vi "电源管理UI.vi"() -> ()   [LabVIEW 2016, in "PLC.lvlib"]
uses:
  PLC.lvlib
  <vilib>/Utility/miscctls.llb/LVPointTypeDef.ctl
  <vilib>/ptbypt/NI_PtbyPt.lvlib
panel:
  in  "副屏看门狗启用":u16(ring) caption="副屏看门狗启用：" items=["关闭", "打开"]
  in  "副屏看门狗设置":u16 caption="副屏看门狗设置："
  out "副屏看门狗计时":u16 caption="副屏看门狗计时："
  in  "主屏看门狗启用":u16(ring) caption="主屏看门狗启用：" items=["关闭", "打开"]
  in  "主屏看门狗设置":u16 caption="主屏看门狗设置："
  out "主屏看门狗计时":u16 caption="主屏看门狗计时："
  out "漏电报警累加值":u16 caption="漏电报警累加值："
  out "外部电源状态":u16(ring) caption="外部电源状态：" items=["正常", "异常"]
  out "当前报警状态":u16(ring) caption="当前报警状态：" items=["无报警"=0, "过压报警"=1, "欠压报警"=2, "过流报警"=4, "漏电报警"=8]
  out "通讯状态":u16(ring) caption="通讯状态：" items=["正常", "异常"]
  out "合闸状态":u16(ring) caption="内部电源状态：" items=["断开", "打开"]
  out "过流报警累加值":u16 caption="过流报警累加值："
  out "欠压报警累加值":u16 caption="欠压报警累加值："
  out "过压报警累加值":u16 caption="过压报警累加值："
  out "当前漏电电流":dbl caption="当前漏电电流："
  out "当前电流":dbl caption="当前电流："
  out "当前电压":u16 caption="当前电压："
  in  "总氮电源":bool
  in  "CODCr电源":bool
  in  "总磷电源":bool
  in  "氨氮电源":bool
  in  "CODMn电源":bool
  in  "多参数电源":bool
  # "s"
  # "s"
  # "s"
  # "s"
  # "mA"
  # "A"
  # "V"
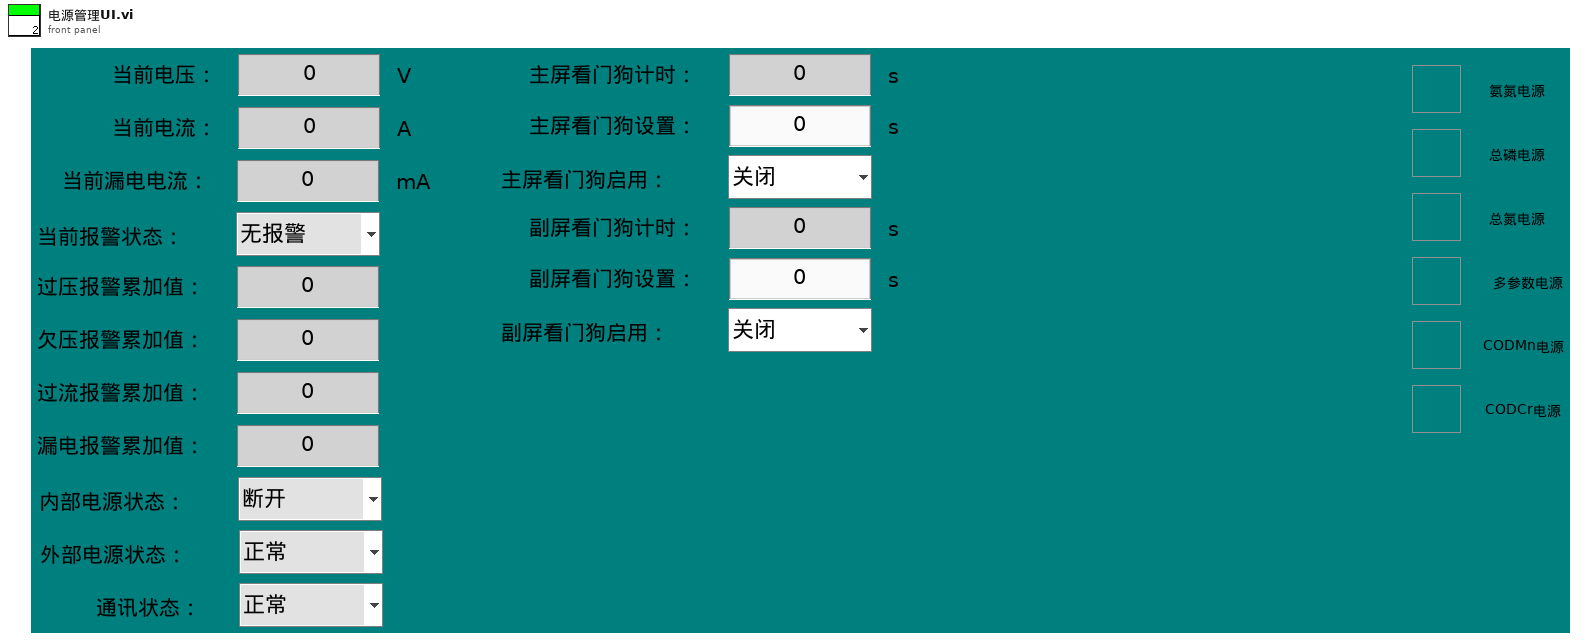
[diagram p1: front panel]
types:
  T1 = typedef "LVPointTypeDef.ctl" = cluster{"Horizontal":i16, "Vertical":i16}
  T2 = cluster{"R0":i16, "R1":i16, "R2":i16, "R3":i16, "R4":i16, "R5":i16, "R6":i16, "R7":i16, "R8":i16, "R9":i16, "R10":i16, "R11":i16, "R12":i16, "R13":i16, "R14":i16, "R15":i16, "R16":i16, "R17":i16, "R18":i16, "R19":i16, "R20":i16, "R21":i16, "R22":i16, "R23":i16, "R24":i16, "R25":i16, "R26":i16, "R27":i16, "R28":i16, "R29":i16, "R30":i16, "R31":i16, "R32":i16, "R33":i16, "R34":i16, "R35":i16, "R36":i16, "R37":i16, "R38":i16, "R39":i16}
  T3 = cluster{"R100":i16, "R101":i16, "R102":i16, "R103":i16, "R104":i16, "R105":i16, "R106":i16, "R107":i16, "R108":i16, "R109":i16, "R110":i16, "R111":i16, "R112":i16, "R113":i16, "R114":i16, "R115":i16, "R116":i16, "R117":i16, "R118":i16, "R119":i16}
  T4 = cluster{"时间标识":timestamp, "设备":string, "日志信息":string}
  T5 = cluster{"命令":string, "数据":cluster{"starting address":u16, "holding register values":u16[]}}
  T6 = cluster{"命令":string, "数据":cluster{"starting address":u16, "holding register value":u16}}
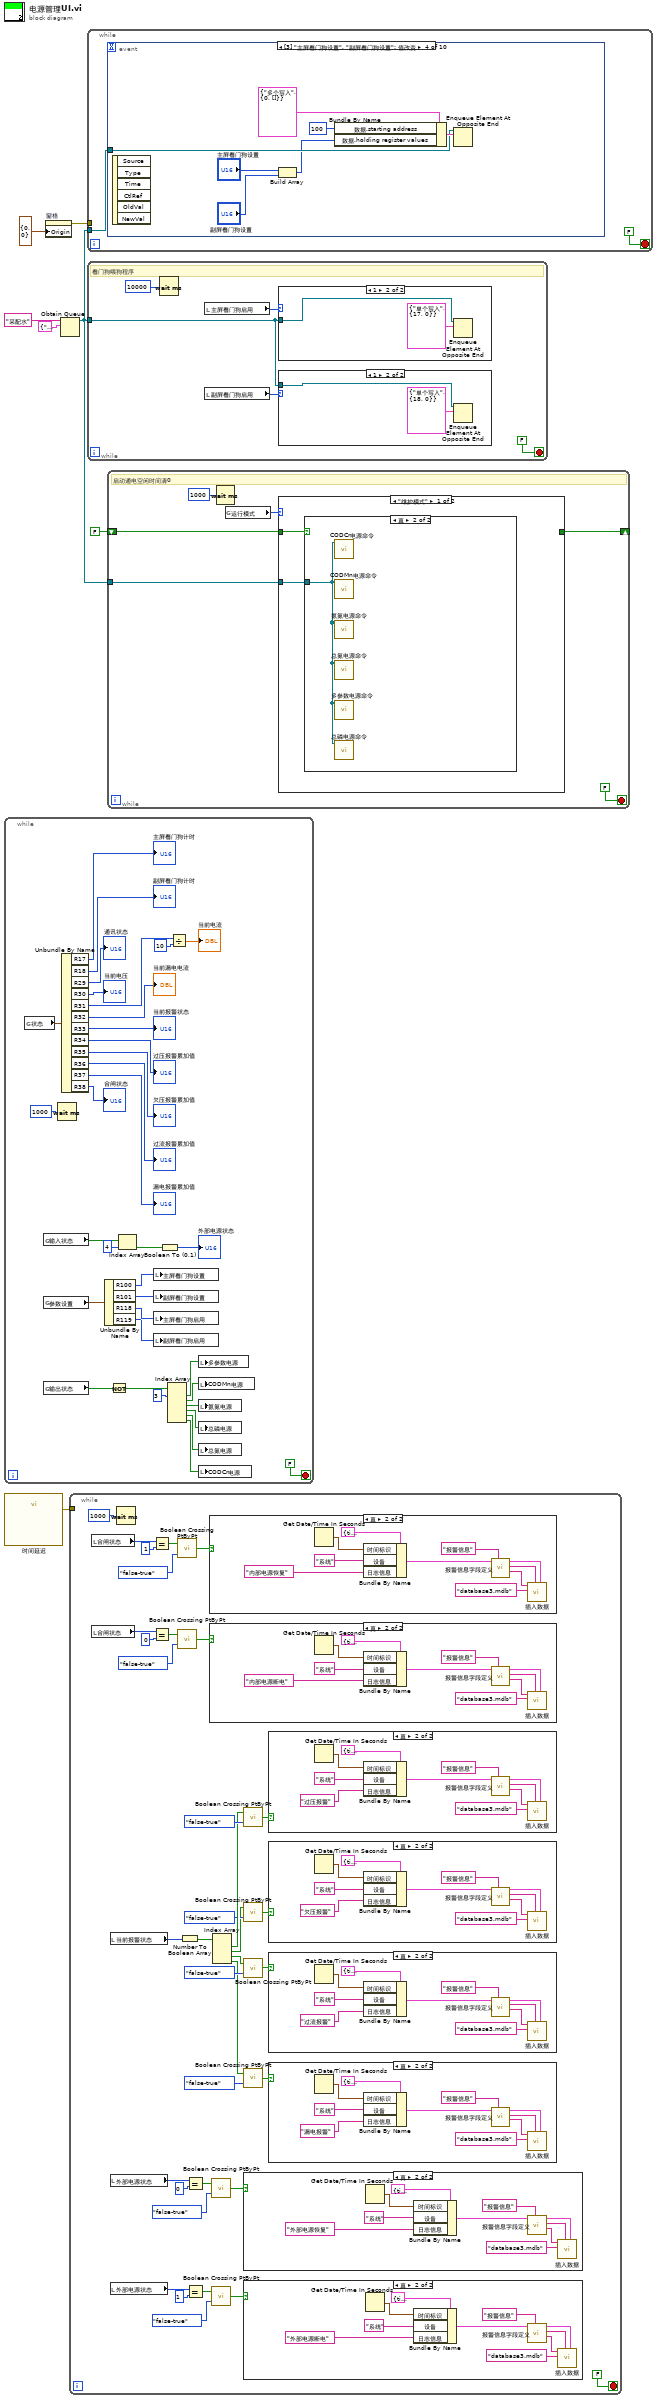
[diagram p0: block diagram]
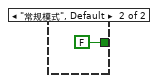
[diagram p13: hidden frame]
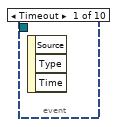
[diagram p14: hidden frame]
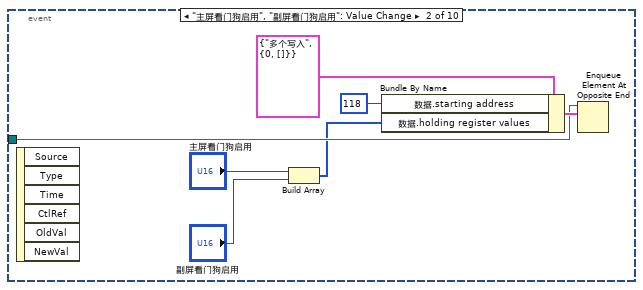
[diagram p15: hidden frame]
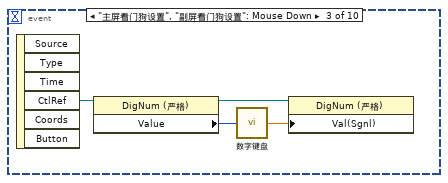
[diagram p16: hidden frame]
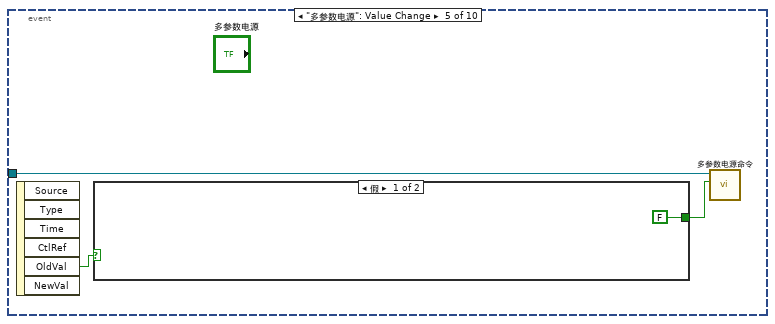
[diagram p17: hidden frame]
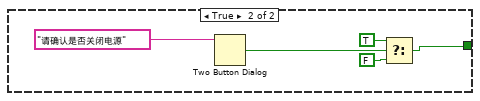
[diagram p18: hidden frame]
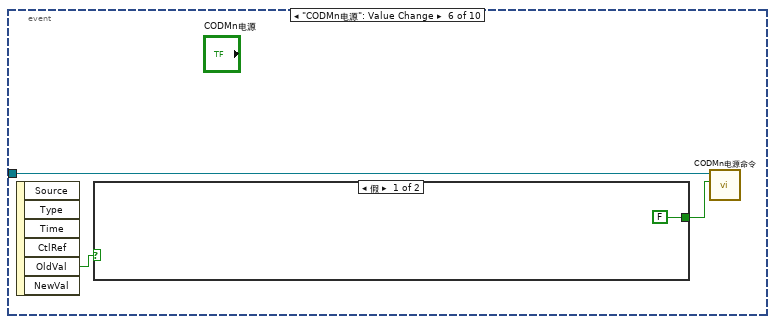
[diagram p19: hidden frame]
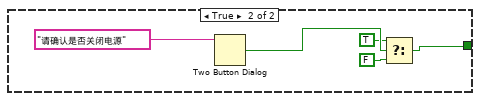
[diagram p20: hidden frame]
diagram:
  n1 = while {
    stop <- FALSE stop-if-true
    n2 = global read "采配水全局变量.vi" "状态"() -> (w31:T2)
    n3 = global read "采配水全局变量.vi" "输入状态"() -> (w18:bool[])
    n4 = global read "采配水全局变量.vi" "参数设置"() -> (w12:T3)
    n5 = global read "采配水全局变量.vi" "输出状态"() -> (w40:bool[])
    n6 = Wait (ms)(milliseconds to wait=u32 1000 ("等待时间（毫秒）")) -> ()  [unwired: 1 out]
    n7 = Unbundle By Name(w31) -> ("R17"=→"主屏看门狗计时":i16, "R18"=→"副屏看门狗计时":i16, "R29"=→"通讯状态":i16, "R30"=→"当前电压":i16, "R31"=w28:i16, "R32"=→"当前漏电电流":i16, "R33"=→"当前报警状态":i16, "R34"=→"过压报警累加值":i16, "R35"=→"欠压报警累加值":i16, "R36"=→"过流报警累加值":i16, "R37"=→"漏电报警累加值":i16, "R38"=→"合闸状态":i16)
    n8 = Unbundle By Name(w12) -> ("R100"=w11:i16, "R101"=w10:i16, "R118"=w9:i16, "R119"=w8:i16)
    n9 = Not(x=w40) -> (.not. x?=w32:bool[])
    n10 = Index Array(array=w18, index=4 ("索引")) -> (element=w16:bool)
    n11 = local write "主屏看门狗设置"(w11) -> ()
    n12 = local write "副屏看门狗设置"(w10) -> ()
    n13 = local write "主屏看门狗启用"(w9) -> ()
    n14 = local write "副屏看门狗启用"(w8) -> ()
    n15 = Boolean To (0,1)(Boolean=w16) -> (0, 1=→"外部电源状态":i16)
    n16 = Index Array(array=w32, index #1=3 ("索引")) -> (element #1=w35:bool, element #2=w38:bool, element #3=w37:bool, element #4=w36:bool, element #5=w34:bool, element #6=w33:bool)  [unwired: 5 in]
    n17 = Divide(x=w28, y=i16 10) -> (x/y=→"当前电流":dbl)
    n18 = local write "多参数电源"(w35) -> ()
    n19 = local write "CODMn电源"(w38) -> ()
    n20 = local write "氨氮电源"(w37) -> ()
    n21 = local write "总磷电源"(w36) -> ()
    n22 = local write "总氮电源"(w34) -> ()
    n23 = local write "CODCr电源"(w33) -> ()
  }
  n24 = call "时间延迟"() -> ("error out"=w2:errorcluster)  [unwired: 11 in]
  n25 = property on="窗格" class="Pane"("Origin"=T1 {"Horizontal"=0, "Vertical"=0} ("原点")) -> (error out=w4:errorcluster)  [unwired: 2 in, 1 out]
  n26 = Obtain Queue(name (unnamed)="采配水" ("名称（未命名）"), element data type=cluster{"命令":string, "数据":variant} {"命令"="", "数据"=variant}) -> (queue out=w1:refnum<queue>)  [unwired: 3 in, 2 out]
  n27 = while {
    tunnel: w2 -> [_]
    stop <- FALSE stop-if-true
    n28 = local read "合闸状态"() -> (w68:u16)
    n29 = local read "合闸状态"() -> (w59:u16)
    n30 = local read "当前报警状态"() -> (w58:u16)
    n31 = local read "外部电源状态"() -> (w78:u16)
    n32 = local read "外部电源状态"() -> (w69:u16)
    n33 = Wait (ms)(milliseconds to wait=u32 1000 ("等待时间（毫秒）")) -> ()  [unwired: 1 out]
    n34 = Equal?(x=w68, y=u16 1) -> (x = y?=w66:bool)
    n35 = Equal?(x=w59, y=u16 0) -> (x = y?=w61:bool)
    n36 = call <vilib>:"Boolean Crossing PtByPt.vi"("direction"=enum16{"either", "false-true", "true-false"}."false-true", "input"=w66) -> ("crossing"=w64:bool)  [unwired: 1 in]
    n37 = call <vilib>:"Boolean Crossing PtByPt.vi"("direction"=enum16{"either", "false-true", "true-false"}."false-true", "input"=w61) -> ("crossing"=w63:bool)  [unwired: 1 in]
    n38 = Number To Boolean Array(number=w58) -> (Boolean array=w57:bool[])
    n39 = Equal?(x=w78, y=u16 0) -> (x = y?=w76:bool)
    n40 = Equal?(x=w69, y=u16 1) -> (x = y?=w71:bool)
    n41 = case shown="真" w64 {
      frame False {
      }
      frame True {
        n42 = Get Date/Time In Seconds() -> (seconds since 1Jan1904=w137:timestamp)
        n43 = Bundle By Name(cluster=T4 {"时间标识"=timestamp(0 s since 1904-01-01), "设备"="", "日志信息"=""} ("data in"), "时间标识"=w137, "设备"="系统", "日志信息"="内部电源恢复") -> (w136:T4)
        n44 = call "报警信息字段定义.vi"("table输入"="报警信息", "data in"=w136) -> ("table输出"=w132:string, "columns"=w131:string[], "data out"=w130:T4)  [unwired: 7 in]
        n45 = call "插入数据.vi"("data"=w130, "columns"=w131, "database"="database3.mdb", "table"=w132) -> ()  [unwired: 7 in, 1 out]
      }
    }
    n46 = case shown="真" w63 {
      frame False {
      }
      frame True {
        n47 = Get Date/Time In Seconds() -> (seconds since 1Jan1904=w127:timestamp)
        n48 = Bundle By Name(cluster=T4 {"时间标识"=timestamp(0 s since 1904-01-01), "设备"="", "日志信息"=""} ("data in"), "时间标识"=w127, "设备"="系统", "日志信息"="内部电源断电") -> (w126:T4)
        n49 = call "报警信息字段定义.vi"("table输入"="报警信息", "data in"=w126) -> ("table输出"=w122:string, "columns"=w121:string[], "data out"=w120:T4)  [unwired: 7 in]
        n50 = call "插入数据.vi"("data"=w120, "columns"=w121, "database"="database3.mdb", "table"=w122) -> ()  [unwired: 7 in, 1 out]
      }
    }
    n51 = call <vilib>:"Boolean Crossing PtByPt.vi"("direction"=enum16{"either", "false-true", "true-false"}."false-true", "input"=w76) -> ("crossing"=w74:bool)  [unwired: 1 in]
    n52 = call <vilib>:"Boolean Crossing PtByPt.vi"("direction"=enum16{"either", "false-true", "true-false"}."false-true", "input"=w71) -> ("crossing"=w73:bool)  [unwired: 1 in]
    n53 = Index Array(array=w57) -> (element #1=w55:bool, element #2=w49:bool, element #3=w48:bool, element #4=w45:bool)  [unwired: 4 in]
    n54 = call <vilib>:"Boolean Crossing PtByPt.vi"("direction"=enum16{"either", "false-true", "true-false"}."false-true", "input"=w55) -> ("crossing"=w54:bool)  [unwired: 1 in]
    n55 = call <vilib>:"Boolean Crossing PtByPt.vi"("direction"=enum16{"either", "false-true", "true-false"}."false-true", "input"=w49) -> ("crossing"=w53:bool)  [unwired: 1 in]
    n56 = call <vilib>:"Boolean Crossing PtByPt.vi"("direction"=enum16{"either", "false-true", "true-false"}."false-true", "input"=w48) -> ("crossing"=w50:bool)  [unwired: 1 in]
    n57 = call <vilib>:"Boolean Crossing PtByPt.vi"("direction"=enum16{"either", "false-true", "true-false"}."false-true", "input"=w45) -> ("crossing"=w47:bool)  [unwired: 1 in]
    n58 = case shown="真" w74 {
      frame False {
      }
      frame True {
        n59 = Get Date/Time In Seconds() -> (seconds since 1Jan1904=w157:timestamp)
        n60 = Bundle By Name(cluster=T4 {"时间标识"=timestamp(0 s since 1904-01-01), "设备"="", "日志信息"=""} ("data in"), "时间标识"=w157, "设备"="系统", "日志信息"="外部电源恢复") -> (w156:T4)
        n61 = call "报警信息字段定义.vi"("table输入"="报警信息", "data in"=w156) -> ("table输出"=w152:string, "columns"=w151:string[], "data out"=w150:T4)  [unwired: 7 in]
        n62 = call "插入数据.vi"("data"=w150, "columns"=w151, "database"="database3.mdb", "table"=w152) -> ()  [unwired: 7 in, 1 out]
      }
    }
    n63 = case shown="真" w73 {
      frame False {
      }
      frame True {
        n64 = Get Date/Time In Seconds() -> (seconds since 1Jan1904=w147:timestamp)
        n65 = Bundle By Name(cluster=T4 {"时间标识"=timestamp(0 s since 1904-01-01), "设备"="", "日志信息"=""} ("data in"), "时间标识"=w147, "设备"="系统", "日志信息"="外部电源断电") -> (w146:T4)
        n66 = call "报警信息字段定义.vi"("table输入"="报警信息", "data in"=w146) -> ("table输出"=w142:string, "columns"=w141:string[], "data out"=w140:T4)  [unwired: 7 in]
        n67 = call "插入数据.vi"("data"=w140, "columns"=w141, "database"="database3.mdb", "table"=w142) -> ()  [unwired: 7 in, 1 out]
      }
    }
    n68 = case shown="真" w54 {
      frame False {
      }
      frame True {
        n69 = Get Date/Time In Seconds() -> (seconds since 1Jan1904=w117:timestamp)
        n70 = Bundle By Name(cluster=T4 {"时间标识"=timestamp(0 s since 1904-01-01), "设备"="", "日志信息"=""} ("data in"), "时间标识"=w117, "设备"="系统", "日志信息"="过压报警") -> (w116:T4)
        n71 = call "报警信息字段定义.vi"("table输入"="报警信息", "data in"=w116) -> ("table输出"=w112:string, "columns"=w111:string[], "data out"=w110:T4)  [unwired: 7 in]
        n72 = call "插入数据.vi"("data"=w110, "columns"=w111, "database"="database3.mdb", "table"=w112) -> ()  [unwired: 7 in, 1 out]
      }
    }
    n73 = case shown="真" w53 {
      frame False {
      }
      frame True {
        n74 = Get Date/Time In Seconds() -> (seconds since 1Jan1904=w107:timestamp)
        n75 = Bundle By Name(cluster=T4 {"时间标识"=timestamp(0 s since 1904-01-01), "设备"="", "日志信息"=""} ("data in"), "时间标识"=w107, "设备"="系统", "日志信息"="欠压报警") -> (w106:T4)
        n76 = call "报警信息字段定义.vi"("table输入"="报警信息", "data in"=w106) -> ("table输出"=w102:string, "columns"=w101:string[], "data out"=w100:T4)  [unwired: 7 in]
        n77 = call "插入数据.vi"("data"=w100, "columns"=w101, "database"="database3.mdb", "table"=w102) -> ()  [unwired: 7 in, 1 out]
      }
    }
    n78 = case shown="真" w50 {
      frame False {
      }
      frame True {
        n79 = Get Date/Time In Seconds() -> (seconds since 1Jan1904=w97:timestamp)
        n80 = Bundle By Name(cluster=T4 {"时间标识"=timestamp(0 s since 1904-01-01), "设备"="", "日志信息"=""} ("data in"), "时间标识"=w97, "设备"="系统", "日志信息"="过流报警") -> (w96:T4)
        n81 = call "报警信息字段定义.vi"("table输入"="报警信息", "data in"=w96) -> ("table输出"=w92:string, "columns"=w91:string[], "data out"=w90:T4)  [unwired: 7 in]
        n82 = call "插入数据.vi"("data"=w90, "columns"=w91, "database"="database3.mdb", "table"=w92) -> ()  [unwired: 7 in, 1 out]
      }
    }
    n83 = case shown="真" w47 {
      frame False {
      }
      frame True {
        n84 = Get Date/Time In Seconds() -> (seconds since 1Jan1904=w87:timestamp)
        n85 = Bundle By Name(cluster=T4 {"时间标识"=timestamp(0 s since 1904-01-01), "设备"="", "日志信息"=""} ("data in"), "时间标识"=w87, "设备"="系统", "日志信息"="漏电报警") -> (w86:T4)
        n86 = call "报警信息字段定义.vi"("table输入"="报警信息", "data in"=w86) -> ("table输出"=w82:string, "columns"=w81:string[], "data out"=w80:T4)  [unwired: 7 in]
        n87 = call "插入数据.vi"("data"=w80, "columns"=w81, "database"="database3.mdb", "table"=w82) -> ()  [unwired: 7 in, 1 out]
      }
    }
  }
  n88 = while {
    tunnel: w1 -> [w159]
    tunnel: w4 -> [_]
    stop <- FALSE stop-if-true
    n89 = event shown="[3] \"主屏看门狗设置\", \"副屏看门狗设置\": 值改变" {
      selector: _ -> [_ _ _ _ _ _ _ _ _ _]
      dyn-events: _ -> [_ _ _ _ _ _ _ _ _ _]
      timeout: _ -> [_ _ _ _ _ _ _ _ _ _]
      tunnel: w159 -> [_ w164 _ w175 w181 w190 w199 w208 w217 w226]
      event Timeout {
        n90 = event-data() -> ()  [unwired: 1 in, 3 out]
      }
      event "主屏看门狗启用", "副屏看门狗启用": Value Change {
        n91 = event-data() -> ()  [unwired: 1 in, 6 out]
        n92 = Build Array("主屏看门狗启用", "副屏看门狗启用") -> (w161:u16[])
        n93 = Bundle By Name(cluster=T5 {"命令"="多个写入", "数据"={"starting address"=0, "holding register values"=[]}} ("元素"), "数据.starting address"=u16 118, "数据.holding register values"=w161) -> (w165:T5)
        n94 = Enqueue Element At Opposite End(queue=w164, element=w165) -> ()  [unwired: 2 in, 3 out]
      }
      event "主屏看门狗设置", "副屏看门狗设置": Mouse Down {
        n95 = event-data() -> ("CtlRef"=w168:refnum<vi>)  [unwired: 1 in, 5 out]
        n96 = property class="DigNum (严格)"(reference=w168) -> (reference out=w170:refnum<vi>, "Value"=w171:u16)  [unwired: 1 in, 1 out]
        n97 = call "数字键盘.vi"("OldNumber"=w171) -> ("NewNumber"=w169:sgl)
        n98 = property class="DigNum (严格)"(reference=w170, "Val(Sgnl)"=w169) -> ()  [unwired: 1 in, 2 out]
      }
      event "主屏看门狗设置", "副屏看门狗设置": Value Change {
        n99 = event-data() -> ()  [unwired: 1 in, 6 out]
        n100 = Build Array("主屏看门狗设置", "副屏看门狗设置") -> (w172:u16[])
        n101 = Bundle By Name(cluster=T5 {"命令"="多个写入", "数据"={"starting address"=0, "holding register values"=[]}} ("元素"), "数据.starting address"=u16 100, "数据.holding register values"=w172) -> (w176:T5)
        n102 = Enqueue Element At Opposite End(queue=w175, element=w176) -> ()  [unwired: 2 in, 3 out]
      }
      event "多参数电源": Value Change {
        n103 = event-data() -> ("OldVal"=w180:bool)  [unwired: 1 in, 5 out]
        n104 = case shown="假" w180 {
          tunnel: [FALSE ("T button?") w183] -> w179
          frame False {
          }
          frame True {
            n105 = Two Button Dialog(message="请确认是否关闭电源" ("消息")) -> (T button?=w186:bool)  [unwired: 2 in]
            n106 = Select(t=TRUE, s=w186, f=FALSE ("T button?")) -> (s? t:f=w183:bool)
          }
        }
        n107 = call "多参数电源命令.vi"("通电/断电"=w179, "队列"=w181) -> ()  [unwired: 9 in, 1 out]
      }
      event "CODMn电源": Value Change {
        n108 = event-data() -> ("OldVal"=w189:bool)  [unwired: 1 in, 5 out]
        n109 = case shown="假" w189 {
          tunnel: [FALSE ("T button?") w192] -> w188
          frame False {
          }
          frame True {
            n110 = Two Button Dialog(message="请确认是否关闭电源" ("消息")) -> (T button?=w195:bool)  [unwired: 2 in]
            n111 = Select(t=TRUE, s=w195, f=FALSE ("T button?")) -> (s? t:f=w192:bool)
          }
        }
        n112 = call "CODMn电源命令.vi"("通电/断电"=w188, "队列"=w190) -> ()  [unwired: 9 in, 1 out]
      }
      event "氨氮电源": Value Change {
        n113 = event-data() -> ("OldVal"=w198:bool)  [unwired: 1 in, 5 out]
        n114 = case shown="假" w198 {
          tunnel: [FALSE ("T button?") w201] -> w197
          frame False {
          }
          frame True {
            n115 = Two Button Dialog(message="请确认是否关闭电源" ("消息")) -> (T button?=w204:bool)  [unwired: 2 in]
            n116 = Select(t=TRUE, s=w204, f=FALSE ("T button?")) -> (s? t:f=w201:bool)
          }
        }
        n117 = call "氨氮电源命令.vi"("通电/断电"=w197, "队列"=w199) -> ()  [unwired: 9 in, 1 out]
      }
      event "总磷电源": Value Change {
        n118 = event-data() -> ("OldVal"=w207:bool)  [unwired: 1 in, 5 out]
        n119 = case shown="假" w207 {
          tunnel: [FALSE ("T button?") w210] -> w206
          frame False {
          }
          frame True {
            n120 = Two Button Dialog(message="请确认是否关闭电源" ("消息")) -> (T button?=w213:bool)  [unwired: 2 in]
            n121 = Select(t=TRUE, s=w213, f=FALSE ("T button?")) -> (s? t:f=w210:bool)
          }
        }
        n122 = call "总磷电源命令.vi"("通电/断电"=w206, "队列"=w208) -> ()  [unwired: 9 in, 1 out]
      }
      event "CODCr电源": Value Change {
        n123 = event-data() -> ("OldVal"=w216:bool)  [unwired: 1 in, 5 out]
        n124 = case shown="假" w216 {
          tunnel: [FALSE ("T button?") w219] -> w215
          frame False {
          }
          frame True {
            n125 = Two Button Dialog(message="请确认是否关闭电源" ("消息")) -> (T button?=w222:bool)  [unwired: 2 in]
            n126 = Select(t=TRUE, s=w222, f=FALSE ("T button?")) -> (s? t:f=w219:bool)
          }
        }
        n127 = call "CODCr电源命令.vi"("通电/断电"=w215, "队列"=w217) -> ()  [unwired: 9 in, 1 out]
      }
      event "总氮电源": Value Change {
        n128 = event-data() -> ("OldVal"=w224:bool)  [unwired: 1 in, 5 out]
        n129 = case shown="假" w224 {
          tunnel: [FALSE ("T button?") w228] -> w225
          frame False {
          }
          frame True {
            n130 = Two Button Dialog(message="请确认是否关闭电源" ("消息")) -> (T button?=w231:bool)  [unwired: 2 in]
            n131 = Select(t=TRUE, s=w231, f=FALSE ("T button?")) -> (s? t:f=w228:bool)
          }
        }
        n132 = call "总氮电源命令.vi"("通电/断电"=w225, "队列"=w226) -> ()  [unwired: 9 in, 1 out]
      }
    }
  }
  n133 = while {
    tunnel: w1 -> [w236]
    stop <- FALSE stop-if-true
    # "看门狗喂狗程序"
    n134 = Wait (ms)(milliseconds to wait=u32 10000 ("等待时间（毫秒）")) -> ()  [unwired: 1 out]
    n135 = local read "主屏看门狗启用"() -> (w235:u16)
    n136 = local read "副屏看门狗启用"() -> (w234:u16)
    n137 = case shown="1" w235 {
      tunnel: w236 -> [_ w240]
      frame 0, Default {
      }
      frame 1 {
        n138 = Enqueue Element At Opposite End(queue=w240, element=T6 {"命令"="单个写入", "数据"={"starting address"=17, "holding register value"=0}} ("元素")) -> ()  [unwired: 2 in, 3 out]
      }
    }
    n139 = case shown="1" w234 {
      tunnel: w236 -> [_ w238]
      frame 0, Default {
      }
      frame 1 {
        n140 = Enqueue Element At Opposite End(queue=w238, element=T6 {"命令"="单个写入", "数据"={"starting address"=18, "holding register value"=0}} ("元素")) -> ()  [unwired: 2 in, 3 out]
      }
    }
  }
  n141 = while {
    tunnel: w1 -> [w245]
    shift-right: [w242] -> _
    shift-left: FALSE -> [w243]
    stop <- FALSE stop-if-true
    # "启动通电空闲时间清0"
    n142 = Wait (ms)(milliseconds to wait=u32 1000 ("等待时间（毫秒）")) -> ()  [unwired: 1 out]
    n143 = global read "系统设置全局变量.vi" "运行模式"() -> (w244:enum16{"维护模式", "常规模式", "应急模式", "质控模式"})
    n144 = case shown="\"维护模式\"" w244 {
      tunnel: w245 -> [w249 _]
      tunnel: w243 -> [w248 _]
      tunnel: [_ FALSE] -> w242
      frame "维护模式" {
        n145 = case shown="真" w248 {
          tunnel: w249 -> [_ w250]
          frame False {
          }
          frame True {
            n146 = call "CODCr电源命令.vi"("队列"=w250) -> ()  [unwired: 10 in, 1 out]
            n147 = call "CODMn电源命令.vi"("队列"=w250) -> ()  [unwired: 10 in, 1 out]
            n148 = call "氨氮电源命令.vi"("队列"=w250) -> ()  [unwired: 10 in, 1 out]
            n149 = call "总氮电源命令.vi"("队列"=w250) -> ()  [unwired: 10 in, 1 out]
            n150 = call "多参数电源命令.vi"("队列"=w250) -> ()  [unwired: 10 in, 1 out]
            n151 = call "总磷电源命令.vi"("队列"=w250) -> ()  [unwired: 10 in, 1 out]
          }
        }
      }
      frame "常规模式", Default {
      }
    }
  }
